vi "kvCanObjBufSetMsgCount.vi"(2 "error in (no error)":errorcluster, 3 "Message Count":u32, 4 "Object Handle":i32, 5 "Channel Handle (input only)":i32) -> (0 "error out":errorcluster, 1 "Channel Handle (output only)":i32)   [LabVIEW 2022 SP3]
doc: "Establishes a maximum number of transmissions to be made by the object buffer."
uses:
  canlib32.dll
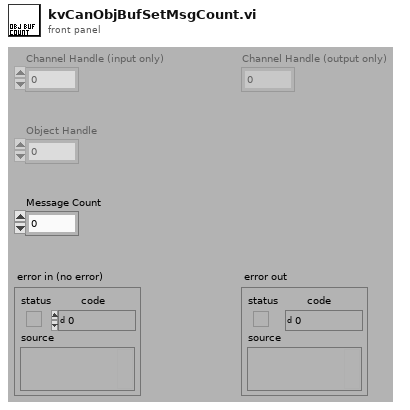
[diagram p1: front panel]
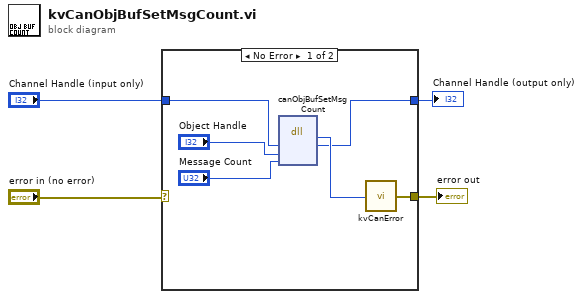
[diagram p0: block diagram]
diagram:
  n1 = case shown="No Error" "error in (no error)" {
    selector: "error in (no error)" -> [_ w12]
    tunnel: [w10 w12] -> w1
    tunnel: "Channel Handle (input only)" -> [w9 w11]
    tunnel: [w5 w11] -> w2
    frame No Error {
      n2 = dll-call lib="canlib32.dll" fn="canObjBufSetMsgCount"("channelHandle"=w9, "objectHandle"="Object Handle", "msgCount"="Message Count") -> (w6:i32, "channelHandle"=w5:i32)  [unwired: 5 in, 2 out]
      n3 = call "kvCanError.vi"("error code"=w6) -> ("error out"=w10:errorcluster)
    }
    frame Error {
    }
  }
  "error out" <- w1
  "Channel Handle (output only)" <- w2
